vi "ni579x Configure RF Filter.vi"(0 "Register Bus":refnum<class "ni579x Register Bus v1 Host.lvclass">=refnum, 1 "scope":string(combo)="rx", 5 "frequency [Hz]":dbl format="%#_6p", 11 "Error In":errorcluster) -> (4 "Register Bus (out)":refnum<class "ni579x Register Bus v1 Host.lvclass">, 6 "coerced frequency [Hz]":dbl format="%#_6p", 15 "Error Out":errorcluster)   [LabVIEW 2015]
uses:
  <instrlib>/ni579x/Register Bus/v1/Host/ni579x Register Bus v1 Host.lvclass
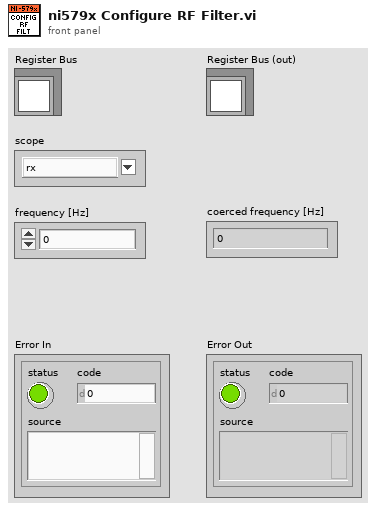
[diagram p1: front panel]
types:
  T1 = typedef "ni579x User Command.ctl" = cluster{"User Data 0":u8, "User Data 1":u8, "User Command ID":T2}
  T2 = typedef "ni579x User Command ID.ctl" = u8
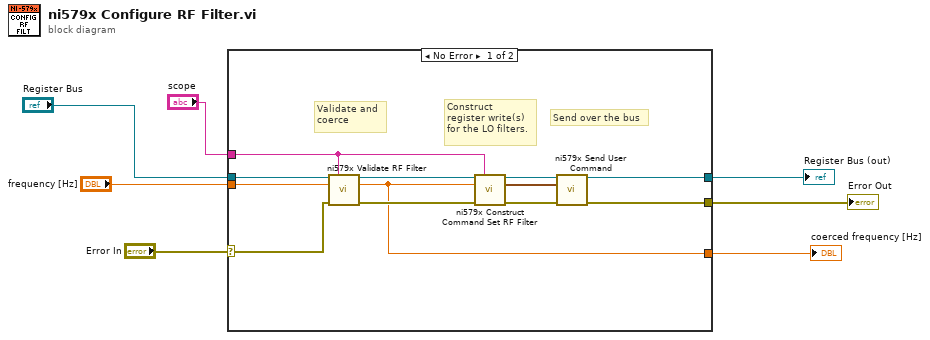
[diagram p0: block diagram]
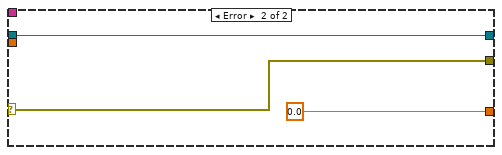
[diagram p2: hidden frame]
diagram:
  n1 = case shown="No Error" "Error In" {
    selector: "Error In" -> [w17 w22]
    tunnel: [w15 w22] -> w6
    tunnel: "Register Bus" -> [w19 w21]
    tunnel: "frequency [Hz]" -> [w18 _]
    tunnel: [w16 w21] -> w3
    tunnel: [w8 0.0 ("coerced attenuation [dB]")] -> w2
    tunnel: "scope" -> [w11 _]
    frame No Error {
      # "Construct\nregister write(s)\nfor the LO filters."
      # "Send over the bus"
      # "Validate and \ncoerce"
      n2 = call <instrlib>:"ni579x Validate RF Filter.vi"("Register Bus"=w19, "scope"=w11, "frequency [Hz]"=w18, "Error In"=w17) -> ("Register Bus (out)"=w10:refnum<class "ni579x Register Bus v1 Host.lvclass">, "coerced frequency [Hz]"=w8:dbl, "Error Out"=w9:errorcluster)  [unwired: 9 in]
      n3 = call <instrlib>:"ni579x Construct Command Set RF Filter.vi"("Register Bus"=w10, "scope"=w11, "frequency [Hz]"=w8, "Error In"=w9) -> ("Register Bus (out)"=w14:refnum<class "ni579x Register Bus v1 Host.lvclass">, "User Command"=w13:T1, "Error Out"=w12:errorcluster)  [unwired: 9 in]
      n4 = call <instrlib>:"ni579x Send User Command.vi"("Register Bus"=w14, "User Command"=w13, "Error In"=w12) -> ("Register Bus (out)"=w16:refnum<class "ni579x Register Bus v1 Host.lvclass">, "Error Out"=w15:errorcluster)  [unwired: 8 in, 3 out]
    }
    frame Error {
    }
  }
  "Register Bus (out)" <- w3
  "Error Out" <- w6
  "coerced frequency [Hz]" <- w2
